vi "Tutorial_8_diff cases.vi"() -> ()   [LabVIEW 2020]
uses:
  Enum_tut8.ctl
panel:
  out "Numeric":i32
  in  "Login UI":enum32{"Page 1"}(tab)
  out "Status":bool
  in  "btnLogin":bool
  in  "Password":string
  in  "User Name":string
  # "Client"
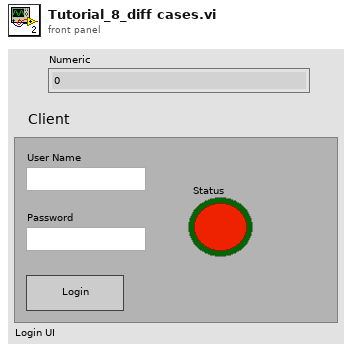
[diagram p1: front panel]
types:
  T1 = typedef "Enum_tut8.ctl" = enum16{"Start", "Idle", "EmptyCheck", "DataTransmission", "Welcom", "End"}
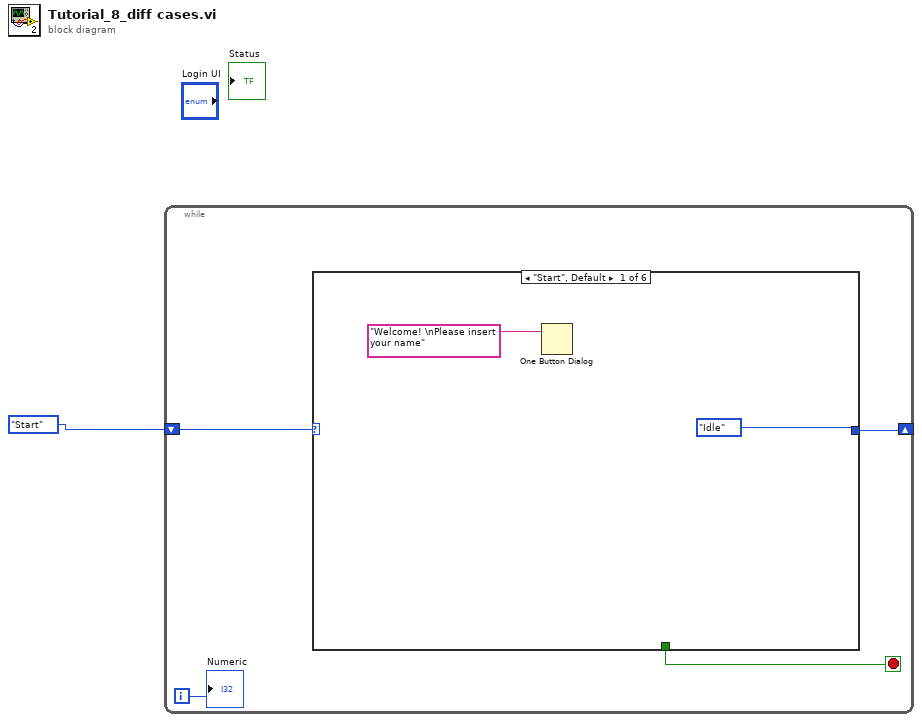
[diagram p0: block diagram]
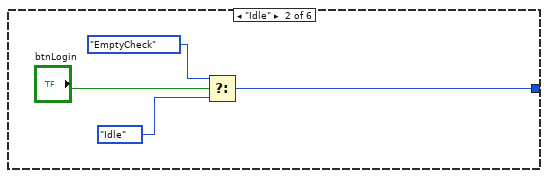
[diagram p2: hidden frame]
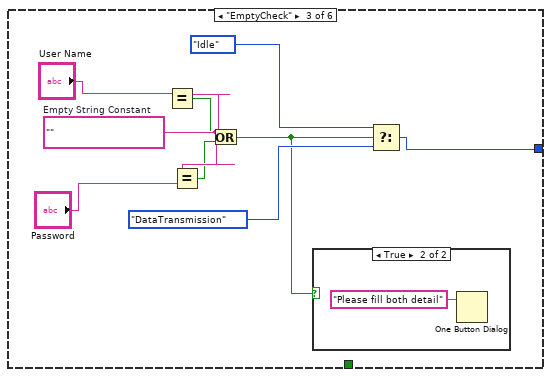
[diagram p3: hidden frame]
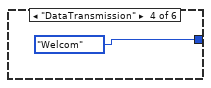
[diagram p5: hidden frame]
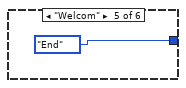
[diagram p6: hidden frame]
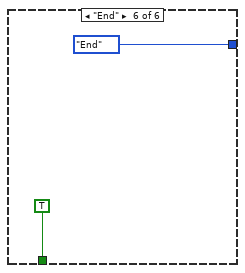
[diagram p7: hidden frame]
diagram:
  n1 = while {
    shift-right: [w2] -> _
    shift-left: Enum_tut8."Start" -> [w5]
    i -> [w3]
    stop <- w4 stop-if-true
    n2 = case shown="\"Start\", Default" w5 {
      tunnel: [_ _ _ _ _ TRUE] -> w4
      tunnel: [Enum_tut8."Idle" w8 w12 Enum_tut8."Welcom" Enum_tut8."End" Enum_tut8."End"] -> w2
      frame "Start", Default {
        n3 = One Button Dialog(message="Welcome! \nPlease insert your name") -> ()  [unwired: 1 in, 1 out]
      }
      frame "Idle" {
        n4 = Select(t=Enum_tut8."EmptyCheck", s="btnLogin", f=Enum_tut8."Idle") -> (s? t:f=w8:T1)
      }
      frame "EmptyCheck" {
        w18 = ""  # Empty String Constant
        n5 = Equal?(x="User Name", y=w18) -> (x = y?=w17:bool)
        n6 = Equal?(x=w18, y="Password") -> (x = y?=w16:bool)
        n7 = Or(x=w17, y=w16) -> (x .or. y?=w13:bool)
        n8 = case shown="True" w13 {
          frame False {
          }
          frame True {
            n9 = One Button Dialog(message="Please fill both detail") -> ()  [unwired: 1 in, 1 out]
          }
        }
        n10 = Select(t=Enum_tut8."Idle", s=w13, f=Enum_tut8."DataTransmission") -> (s? t:f=w12:T1)
      }
      frame "DataTransmission" {
      }
      frame "Welcom" {
      }
      frame "End" {
      }
    }
    "Numeric" <- w3
  }
